vi "EXECUTE SWERVE DRIVE.vi"(0 "Swerve refs":cluster{"Driver":T1, "Steer":T1, "Encoder":T6}[](array[cluster]), 5 "HEADING":dbl, 7 "DRIVE MAX SPEED":dbl=0.7, 9 "STEER MAX speed":dbl=0.7) -> (4 "VELOCITIES":dbl[](array[numeric]), 6 "STEERING\nANGLES (deg)":dbl[](array[numeric]))   [LabVIEW 2023]
uses:
  Global odometry.vi
  Global INIT.vi
  <vilib>/Rock Robotics/SystemInterfaces/DIO/FPGA_DIOPWMChannel.ctl
  <vilib>/Rock Robotics/WPI/PWM/WPI_PWMDeadband.ctl
  <vilib>/Rock Robotics/WPI/MotorControl/WPI_MotorControlType.ctl
  <vilib>/Rock Robotics/SystemInterfaces/DIO/FPGA_DIOChannel.ctl
  <vilib>/Rock Robotics/WPI/MotorControl/WPI_MotorControlDeviceRef.ctl
  <vilib>/Rock Robotics/WPI/ThirdParty/Phoenix-LabVIEW/CANCoder/Controls/CTRE_Phoenix_CANcoder_DeviceRef.ctl
panel:
  out "error out":errorcluster
  in  "error in (no error)":errorcluster
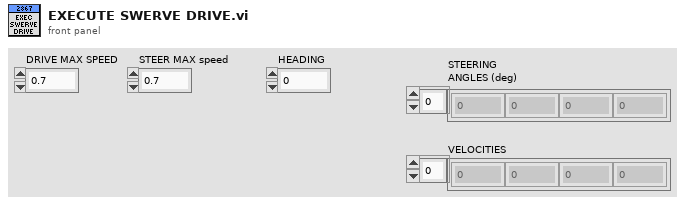
[diagram p1: front panel]
types:
  T1 = typedef "WPI_MotorControlDeviceRef.ctl" = cluster{"DeviceStatus":errorcluster, "Type":T2, "PWM":cluster{"PWM Channel":T3, "DeadBand":T4}, "CAN":cluster{"Device Number":u8, "SetOutput VI Ref":variant, "GetOutput VI Ref":variant, "Enable VI Ref":variant, "Disable VI Ref":variant, "Data":variant}, "Invert":bool, "DIO PWM":cluster{"PWM \"Enable\" Channel":T3, "DIOChannel":T5, "PWM Rate":dbl}}
  T2 = typedef "WPI_MotorControlType.ctl" = enum16{"PWM", "CAN", "DIO PWM"}
  T3 = typedef "FPGA_DIOPWMChannel.ctl" = enum8{"PWM 0", "PWM 1", "PWM 2", "PWM 3", "PWM 4", "PWM 5", "PWM 6", "PWM 7", "PWM 8", "PWM 9", "PWM MXP 0", "PWM MXP 1", "PWM MXP 2", "PWM MXP 3", "PWM MXP 4", "PWM MXP 5", "PWM MXP 6", "PWM MXP 7", "PWM MXP 8", "PWM MXP 9", "Invalid"}
  T4 = typedef "WPI_PWMDeadband.ctl" = cluster{"Name":string, "maxPositivePwm":i32, "minPositivePwm":i32, "centerPwm":i32, "maxNegativePwm":i32, "minNegativePwm":i32, "angularRange":u16}
  T5 = typedef "FPGA_DIOChannel.ctl" = enum8{"DIO 0", "DIO 1", "DIO 2", "DIO 3", "DIO 4", "DIO 5", "DIO 6", "DIO 7", "DIO 8", "DIO 9", "DIO MXP 0", "DIO MXP 1", "DIO MXP 2", "DIO MXP 3", "DIO MXP 4", "DIO MXP 5", "DIO MXP 6", "DIO MXP 7", "DIO MXP 8", "DIO MXP 9", "DIO MXP 10", "DIO MXP 11", "DIO MXP 12", "DIO MXP 13", "DIO MXP 14", "DIO MXP 15", "SPI Port CS1", "SPI Port CS2", "SPI Port CS3", "SPI Port MISO", "SPI Port MOSI", "Invalid"}
  T6 = typedef "CTRE_Phoenix_CANcoder_DeviceRef.ctl" = cluster{"DeviceStatus":errorcluster, "Device Number":u8, "Handle":u64, "UsageFrame":u32, "Library Path":path}
  T7 = typedef "ctrl pivot select.ctl" = enum16{"geometric center", "CG", "FL", "FR", "RR", "RL", "other"}
  T8 = typedef "ctrl XY coord.ctl" = cluster{"X":dbl, "Y":dbl}
  T9 = typedef "ctrl driver input.ctl" = cluster{"Jx":dbl, "Jy":dbl, "Jr ":dbl, "R":dbl, "theta (deg)":dbl, "theta (rad)":dbl, "PARK":bool}
  T10 = typedef "ctrl DRIVING FRAME selector.ctl" = enum16{"ROBO-centric", "FLD-centric"}
  T11 = typedef "ctrl FRONT FACE selector.ctl" = enum16{"intake side", "shooter side"}
  T12 = typedef "WPI_DriverStationAllianceInfo.ctl" = enum16{"Red", "Blue", "Invalid"}
  T13 = typedef "ctrl swerve motor.ctl" = cluster{"description":string, "MOTOR SELECT":T14, "Installed?":bool, "CAN ID":u8, "refnum name":string, "Invert":bool, "Idle Mode":T15, "Current limiting":T16, "MOTOR PIDF coefficients":T17, "gear ratio":dbl}
  T14 = typedef "ctrl MOTOR SELECT.ctl" = i16
  T15 = typedef "Spark MAX Idle Mode.ctl" = enum16{"Coast", "Brake"}
  T16 = typedef "ctrl Spark MAX current limiting.ctl" = cluster{"Linearized":bool, "Free Speed (A)":dbl, "Primay (A)":dbl, "Limit RPM (0)":u32}
  T17 = typedef "ctrl motor PIDF coefficients.ctl" = cluster{"PIDF":cluster{"P Gain":dbl, "I Gain":dbl, "D Gain":dbl, "F Gain":dbl, "I Zone":dbl, "Min Output":dbl, "Max Output":dbl}, "Smart Motion":T18}
  T18 = typedef "Spark MAX Smart Motion Parameters.ctl" = cluster{"Max Velocity":dbl, "Max Acceleration":dbl, "Minimum Velocity Output":dbl, "Allowed Closed Loop Error":dbl}
  T19 = typedef "ctrl Talon FX config.ctl" = cluster{"refnum name":string, "CAN ID":u8, "Installed?":bool, "description":string, "MOTOR SELECT":T14, "CAN Bus":string, "Invert Type":T20, "Neutral Mode":T21, "gear ratio":dbl, "MOTOR PIDF coefficients":T17, "Throttle":cluster{"Ramp Open (s)":dbl, "Ramp Closed (s)":dbl, "Percent Deadband":dbl}, "Supply Current Limits":cluster{"Enable?":bool, "Current Limit":dbl, "Threshold Current":dbl, "Threshold Time":dbl}}
  T20 = typedef "CTRE_Phoenix_MotorControl_TalonFXInvertType.ctl" = enum16{"Counter-Clockwise", "Clockwise"}
  T21 = typedef "CTRE_Phoenix_MotorControl_NeutralMode.ctl" = enum8{"EEPROMSetting", "Override to Coast", "Override to Brake"}
  T22 = typedef "ctrl swerve module.ctl" = cluster{"descr":string, "V":dbl, "POS":dbl, "target":dbl, "ABS":dbl, "from pivot to module":cluster{"R":dbl, "theta (deg)":dbl, "theta spin (deg)":dbl, "theta park (deg)":dbl}, "coord wrt geom CTR":cluster{"X":dbl, "Y":dbl}, "corner wt (lbm)":dbl}
  T23 = enum16{"FRONT RIGHT", "FRONT LEFT", "REAR LEFT", "REAR RIGHT"}
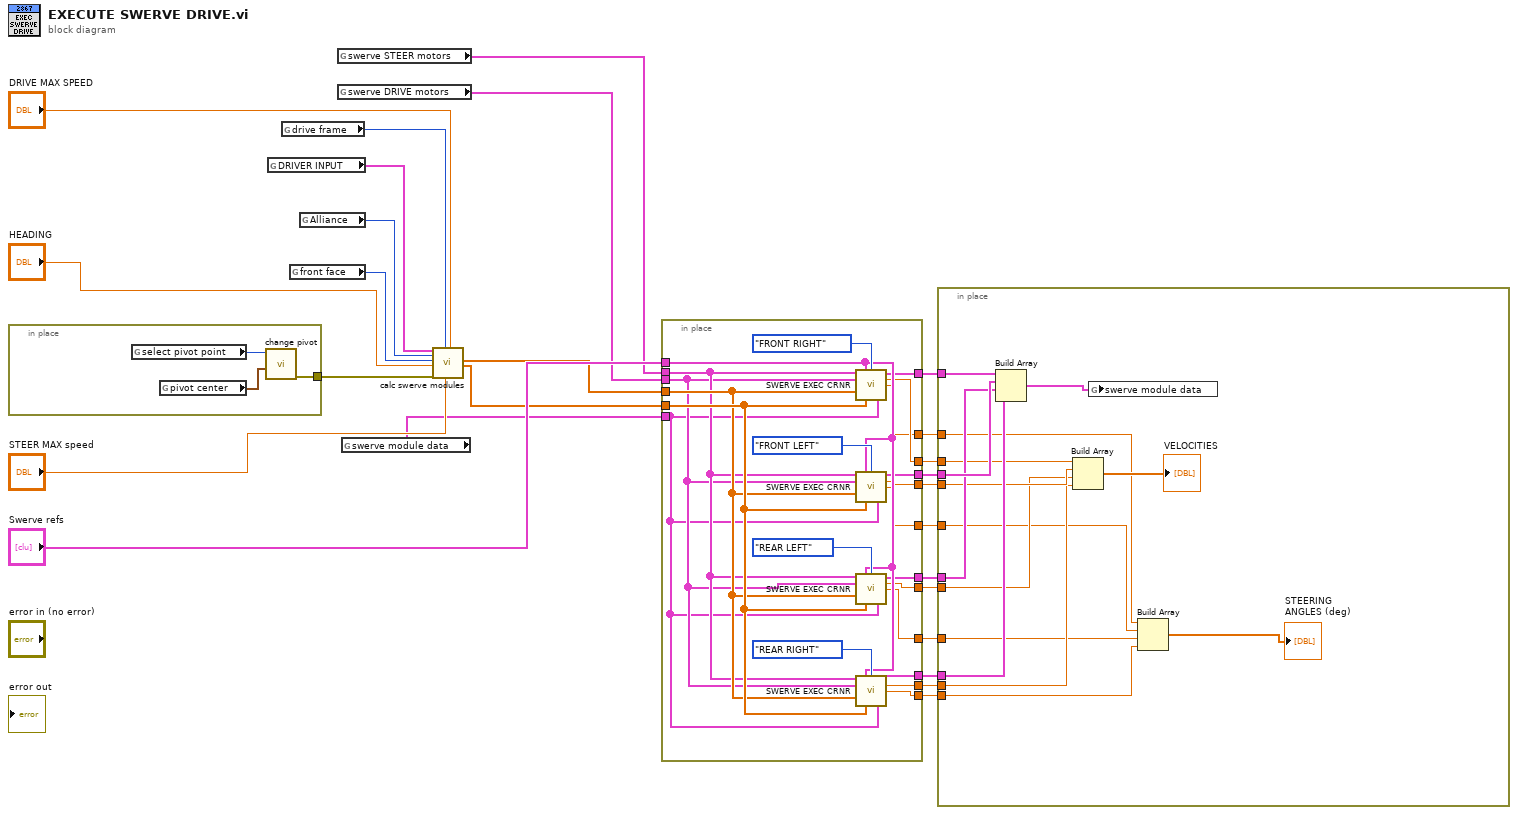
[diagram p0: block diagram]
diagram:
  n1 = in-place {
    in-place-border: [w27] -> w19
    n2 = global read "Global odometry.vi" "select pivot point"() -> (w29:T7)
    n3 = global read "Global odometry.vi" "pivot center"() -> (w28:T8)
    n4 = call "change pivot.vi"("new pivot center"=w28, "select pivot point"=w29) -> ("error out"=w27:errorcluster)  [unwired: 9 in]
  }
  n5 = global read "Global odometry.vi" "DRIVER INPUT"() -> (w20:T9)
  n6 = global read "Global odometry.vi" "drive frame"() -> (w23:T10)
  n7 = global read "Global odometry.vi" "front face"() -> (w21:T11)
  n8 = global read "Global odometry.vi" "Alliance"() -> (w22:T12)
  n9 = global read "Global INIT.vi" "swerve STEER motors"() -> (w15:T13[])
  n10 = global read "Global INIT.vi" "swerve DRIVE motors"() -> (w14:T19[])
  n11 = global read "Global odometry.vi" "swerve module data"() -> (w13:T22[])
  n12 = call "calc swerve modules.vi"("DRIVER INPUT"=w20, "Alliance"=w22, "front face"=w21, "HDG (deg)"="HEADING", "error in (no error)"=w19, "drive frame"=w23, "MAX spin (rev/s)"="STEER MAX speed", "Vmax"="DRIVE MAX SPEED") -> ("speed norm"=w16:dbl[], "angle"=w17:dbl[])  [unwired: 9 in, 1 out]
  n13 = in-place {
    in-place-border: "Swerve refs" -> [w47]
    in-place-border: w17 -> [w46]
    in-place-border: w16 -> [w45]
    in-place-border: w15 -> [w44]
    in-place-border: w14 -> [w43]
    in-place-border: w13 -> [w42]
    in-place-border: [w41] -> w12
    in-place-border: [w40] -> w11
    in-place-border: [w39] -> w10
    in-place-border: [w38] -> w9
    in-place-border: [w37] -> w8
    in-place-border: [w36] -> w7
    in-place-border: [w35] -> w6
    in-place-border: [w34] -> w5
    in-place-border: [w33] -> w4
    in-place-border: [w32] -> w3
    in-place-border: [w31] -> w2
    in-place-border: [w30] -> w1
    n14 = call "SWERVE EXEC CRNR.vi"("swerve STEER motors"=w44, "Swerve refs"=w47, "Swerve position"=T23."FRONT RIGHT", "swerve DRIVE motors"=w43, "speed norm"=w45, "angle"=w46, "swerve module data"=w42) -> ("swerve module out"=w41:T22, "velocity out"=w37:dbl, "steer angle out\n(deg)"=w33:dbl)  [unwired: 6 in]
    n15 = call "SWERVE EXEC CRNR.vi"("swerve STEER motors"=w44, "Swerve refs"=w47, "Swerve position"=T23."FRONT LEFT", "swerve DRIVE motors"=w43, "speed norm"=w45, "angle"=w46, "swerve module data"=w42) -> ("swerve module out"=w40:T22, "velocity out"=w36:dbl, "steer angle out\n(deg)"=w32:dbl)  [unwired: 6 in]
    n16 = call "SWERVE EXEC CRNR.vi"("swerve STEER motors"=w44, "Swerve refs"=w47, "Swerve position"=T23."REAR LEFT", "swerve DRIVE motors"=w43, "speed norm"=w45, "angle"=w46, "swerve module data"=w42) -> ("swerve module out"=w39:T22, "velocity out"=w35:dbl, "steer angle out\n(deg)"=w31:dbl)  [unwired: 6 in]
    n17 = call "SWERVE EXEC CRNR.vi"("swerve STEER motors"=w44, "Swerve refs"=w47, "Swerve position"=T23."REAR RIGHT", "swerve DRIVE motors"=w43, "speed norm"=w45, "angle"=w46, "swerve module data"=w42) -> ("swerve module out"=w38:T22, "velocity out"=w34:dbl, "steer angle out\n(deg)"=w30:dbl)  [unwired: 6 in]
  }
  n18 = in-place {
    in-place-border: w12 -> [w66]
    in-place-border: w11 -> [w65]
    in-place-border: w10 -> [w64]
    in-place-border: w9 -> [w63]
    in-place-border: w8 -> [w61]
    in-place-border: w7 -> [w60]
    in-place-border: w6 -> [w59]
    in-place-border: w5 -> [w58]
    in-place-border: w4 -> [w56]
    in-place-border: w3 -> [w55]
    in-place-border: w2 -> [w54]
    in-place-border: w1 -> [w53]
    n19 = Build Array(w66, w65, w64, w63) -> (w62:T22[])
    n20 = Build Array(w61, w60, w59, w58) -> (→"VELOCITIES":dbl[])
    n21 = global write "Global odometry.vi" "swerve module data"(w62) -> ()
    n22 = Build Array(w56, w55, w54, w53) -> (→"STEERING\nANGLES (deg)":dbl[])
  }
